vi "FTP_QUIT.vi"(0 "connection ID":refnum<k5>, 1 "error in":errorcluster) -> (3 "reply string":string, 4 "Good Reply?":bool, 5 "error out":errorcluster)   [LabVIEW 2012]
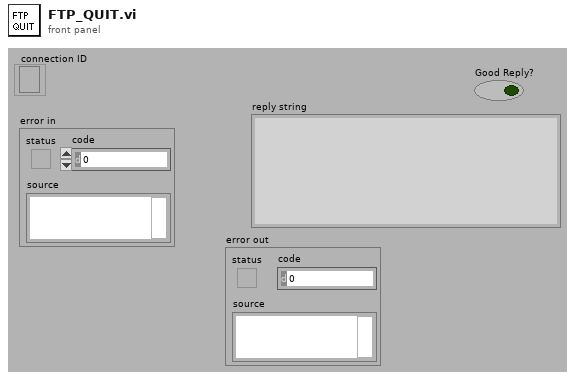
[diagram p1: front panel]
types:
  T1 = enum16{"unknown", "100 + Prelim", "200 + ", "300 + Intermed", "400 - Transient", "500 - Permanent"}
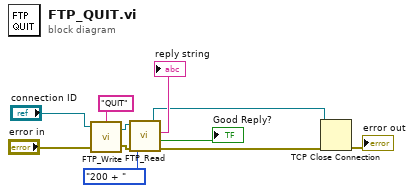
[diagram p0: block diagram]
diagram:
  n1 = call <userlib>:"FTP_Write.vi"("Cmd"="QUIT", "error in"="error in", "connection ID in"="connection ID") -> ("error out"=w7:errorcluster, "connection ID out"=w6:refnum<k5>)  [unwired: 1 in]
  n2 = call <userlib>:"FTP_Read.vi"("error In"=w7, "expected class"=T1."200 + ", "connection ID"=w6) -> ("error out"=w4:errorcluster, "Good Reply?"=→"Good Reply?":bool, "reply string"=→"reply string":string, "connection ID out"=w5:refnum<k5>)  [unwired: 1 out]
  n3 = TCP Close Connection(connection ID=w5, error in (no error)=w4) -> (error out=→"error out":errorcluster)  [unwired: 2 out]
